vi "Individual Tube ON - OFF.vi"(6 "Single Tube ON/OFF":bool, 7 "Tube #":i32 min=0 max=63) -> ()   [LabVIEW 2020]
uses:
  <vilib>/DAQmx/write.llb/DAQmx Write (Digital U8 1Chan 1Samp).vi
  <vilib>/DAQmx/create/channels.llb/DAQmx Create Channel (DO-Digital Output).vi
  <vilib>/DAQmx/miscellaneous.llb/DAQmx Fill In Error Info.vi
panel:
  out "Status(U8) 2":u8
  out "Status(U8)":u8
  in  "lines":tag="Dev2/port0/line0:7"
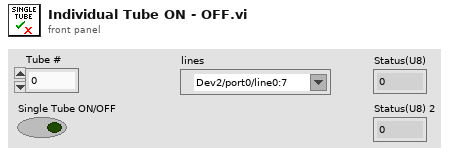
[diagram p1: front panel]
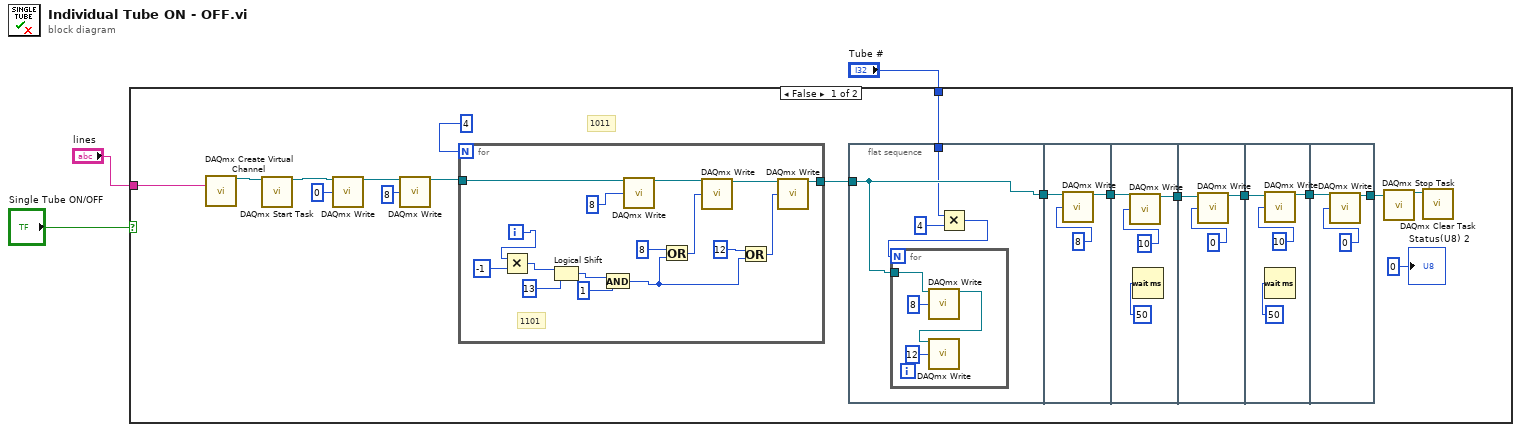
[diagram p0: block diagram]
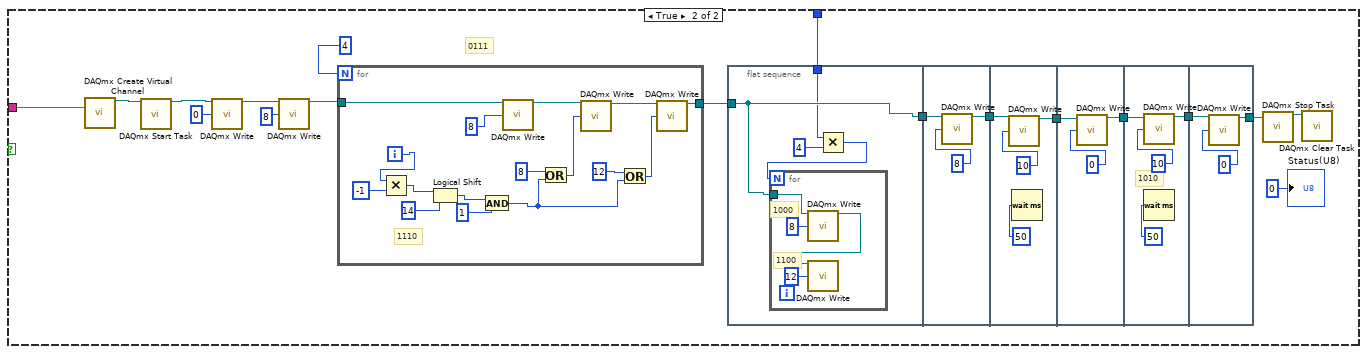
[diagram p2: hidden frame]
diagram:
  n1 = case shown="False" "Single Tube ON/OFF" {
    tunnel: "Tube #" -> [w5 w64]
    tunnel: "lines" -> [w4 w63]
    frame False {
      # "1011"
      n2 = call-poly <vilib>:"DAQmx Create Virtual Channel.vi"("lines"=w4) -> ("task out"=w16:refnum<k21>)  [unwired: 13 in, 1 out]
      n3 = call <vilib>:"DAQmx Start Task.vi"("task/channels in"=w16) -> ("task out"=w11:refnum<k21>)  [unwired: 13 in, 1 out]
      n4 = call-poly <vilib>:"DAQmx Write.vi"("task/channels in"=w11, "data"=u8 0) -> ("task out"=w10:refnum<k21>)  [unwired: 11 in, 2 out]
      n5 = call-poly <vilib>:"DAQmx Write.vi"("task/channels in"=w10, "data"=u8 8) -> ("task out"=w13:refnum<k21>)  [unwired: 11 in, 2 out]
      n6 = for {
        N: 4 -> [_]
        tunnel: w13 -> [w51]
        tunnel: [w48] -> w7
        i -> [w60]
        # "1101"
        n7 = Multiply(x=w60, y=-1) -> (x*y=w58:i32)
        n8 = Logical Shift(y=w58, x=u8 13) -> (x << y=w62:u8)
        n9 = And(x=w62, y=u32 1) -> (x .and. y?=w54:u32)
        n10 = call-poly <vilib>:"DAQmx Write.vi"("task/channels in"=w51, "data"=u32 8 ("x")) -> ("task out"=w50:refnum<k21>)  [unwired: 11 in, 2 out]
        n11 = Or(x=u32 8, y=w54) -> (x .or. y?=w55:u32)
        n12 = call-poly <vilib>:"DAQmx Write.vi"("task/channels in"=w50, "data"=w55) -> ("task out"=w49:refnum<k21>)  [unwired: 11 in, 2 out]
        n13 = Or(x=u32 12, y=w54) -> (x .or. y?=w52:u32)
        n14 = call-poly <vilib>:"DAQmx Write.vi"("task/channels in"=w49, "data"=w52) -> ("task out"=w48:refnum<k21>)  [unwired: 11 in, 2 out]
      }
      n15 = flat-sequence {
        tunnel: [w23] -> w21
        tunnel: w7 -> [w23]
        tunnel: w5 -> [w22]
        tunnel: [w30] -> w20
        tunnel: w21 -> [w31]
        tunnel: w20 -> [w34]
        tunnel: [w33] -> w19
        tunnel: w19 -> [w38]
        tunnel: [w37] -> w18
        tunnel: w18 -> [w41]
        tunnel: [w40] -> w17
        tunnel: w17 -> [w45]
        tunnel: [w44] -> w8
        frame #0 {
          n16 = Multiply(x=w22, y=4) -> (x*y=w25:i32)
          n17 = for {
            N: w25 -> [_]
            tunnel: w23 -> [w27]
            n18 = call-poly <vilib>:"DAQmx Write.vi"("task/channels in"=w27, "data"=u8 8) -> ("task out"=w26:refnum<k21>)  [unwired: 11 in, 2 out]
            n19 = call-poly <vilib>:"DAQmx Write.vi"("task/channels in"=w26, "data"=u8 12) -> ()  [unwired: 11 in, 3 out]
          }
        }
        frame #1 {
          n20 = call-poly <vilib>:"DAQmx Write.vi"("task/channels in"=w31, "data"=u8 8) -> ("task out"=w30:refnum<k21>)  [unwired: 11 in, 2 out]
        }
        frame #2 {
          n21 = call-poly <vilib>:"DAQmx Write.vi"("task/channels in"=w34, "data"=u8 10) -> ("task out"=w33:refnum<k21>)  [unwired: 11 in, 2 out]
          n22 = Wait (ms)(milliseconds to wait=u32 50) -> ()  [unwired: 1 out]
        }
        frame #3 {
          n23 = call-poly <vilib>:"DAQmx Write.vi"("task/channels in"=w38, "data"=u8 0) -> ("task out"=w37:refnum<k21>)  [unwired: 11 in, 2 out]
        }
        frame #4 {
          n24 = call-poly <vilib>:"DAQmx Write.vi"("task/channels in"=w41, "data"=u8 10) -> ("task out"=w40:refnum<k21>)  [unwired: 11 in, 2 out]
          n25 = Wait (ms)(milliseconds to wait=u32 50) -> ()  [unwired: 1 out]
        }
        frame #5 {
          n26 = call-poly <vilib>:"DAQmx Write.vi"("task/channels in"=w45, "data"=u8 0) -> ("task out"=w44:refnum<k21>)  [unwired: 11 in, 2 out]
        }
      }
      n27 = call <vilib>:"DAQmx Stop Task.vi"("task/channels in"=w8) -> ("task out"=w15:refnum<k21>)  [unwired: 13 in, 1 out]
      n28 = call <vilib>:"DAQmx Clear Task.vi"("task in"=w15) -> ()  [unwired: 14 in, 1 out]
      "Status(U8) 2" <- u8 0
    }
    frame True {
      # "0111"
      n29 = call-poly <vilib>:"DAQmx Create Virtual Channel.vi"("lines"=w63) -> ("task out"=w75:refnum<k21>)  [unwired: 13 in, 1 out]
      n30 = call <vilib>:"DAQmx Start Task.vi"("task/channels in"=w75) -> ("task out"=w70:refnum<k21>)  [unwired: 13 in, 1 out]
      n31 = call-poly <vilib>:"DAQmx Write.vi"("task/channels in"=w70, "data"=u8 0) -> ("task out"=w69:refnum<k21>)  [unwired: 11 in, 2 out]
      n32 = call-poly <vilib>:"DAQmx Write.vi"("task/channels in"=w69, "data"=u8 8) -> ("task out"=w72:refnum<k21>)  [unwired: 11 in, 2 out]
      n33 = for {
        N: 4 -> [_]
        tunnel: w72 -> [w110]
        tunnel: [w107] -> w66
        i -> [w119]
        # "1110"
        n34 = Multiply(x=w119, y=-1) -> (x*y=w117:i32)
        n35 = Logical Shift(y=w117, x=u8 14) -> (x << y=w121:u8)
        n36 = And(x=w121, y=u32 1) -> (x .and. y?=w113:u32)
        n37 = call-poly <vilib>:"DAQmx Write.vi"("task/channels in"=w110, "data"=u32 8 ("x")) -> ("task out"=w109:refnum<k21>)  [unwired: 11 in, 2 out]
        n38 = Or(x=u32 8, y=w113) -> (x .or. y?=w114:u32)
        n39 = call-poly <vilib>:"DAQmx Write.vi"("task/channels in"=w109, "data"=w114) -> ("task out"=w108:refnum<k21>)  [unwired: 11 in, 2 out]
        n40 = Or(x=u32 12, y=w113) -> (x .or. y?=w111:u32)
        n41 = call-poly <vilib>:"DAQmx Write.vi"("task/channels in"=w108, "data"=w111) -> ("task out"=w107:refnum<k21>)  [unwired: 11 in, 2 out]
      }
      n42 = flat-sequence {
        tunnel: [w82] -> w80
        tunnel: w66 -> [w82]
        tunnel: w64 -> [w81]
        tunnel: [w89] -> w79
        tunnel: w80 -> [w90]
        tunnel: w79 -> [w93]
        tunnel: [w92] -> w78
        tunnel: w78 -> [w97]
        tunnel: [w96] -> w77
        tunnel: w77 -> [w100]
        tunnel: [w99] -> w76
        tunnel: w76 -> [w104]
        tunnel: [w103] -> w67
        frame #0 {
          n43 = Multiply(x=w81, y=4) -> (x*y=w84:i32)
          n44 = for {
            N: w84 -> [_]
            tunnel: w82 -> [w86]
            # "1100"
            # "1000"
            n45 = call-poly <vilib>:"DAQmx Write.vi"("task/channels in"=w86, "data"=u8 8) -> ("task out"=w85:refnum<k21>)  [unwired: 11 in, 2 out]
            n46 = call-poly <vilib>:"DAQmx Write.vi"("task/channels in"=w85, "data"=u8 12) -> ()  [unwired: 11 in, 3 out]
          }
        }
        frame #1 {
          n47 = call-poly <vilib>:"DAQmx Write.vi"("task/channels in"=w90, "data"=u8 8) -> ("task out"=w89:refnum<k21>)  [unwired: 11 in, 2 out]
        }
        frame #2 {
          n48 = call-poly <vilib>:"DAQmx Write.vi"("task/channels in"=w93, "data"=u8 10) -> ("task out"=w92:refnum<k21>)  [unwired: 11 in, 2 out]
          n49 = Wait (ms)(milliseconds to wait=u32 50) -> ()  [unwired: 1 out]
        }
        frame #3 {
          n50 = call-poly <vilib>:"DAQmx Write.vi"("task/channels in"=w97, "data"=u8 0) -> ("task out"=w96:refnum<k21>)  [unwired: 11 in, 2 out]
        }
        frame #4 {
          # "1010"
          n51 = call-poly <vilib>:"DAQmx Write.vi"("task/channels in"=w100, "data"=u8 10) -> ("task out"=w99:refnum<k21>)  [unwired: 11 in, 2 out]
          n52 = Wait (ms)(milliseconds to wait=u32 50) -> ()  [unwired: 1 out]
        }
        frame #5 {
          n53 = call-poly <vilib>:"DAQmx Write.vi"("task/channels in"=w104, "data"=u8 0) -> ("task out"=w103:refnum<k21>)  [unwired: 11 in, 2 out]
        }
      }
      n54 = call <vilib>:"DAQmx Stop Task.vi"("task/channels in"=w67) -> ("task out"=w74:refnum<k21>)  [unwired: 13 in, 1 out]
      n55 = call <vilib>:"DAQmx Clear Task.vi"("task in"=w74) -> ()  [unwired: 14 in, 1 out]
      "Status(U8)" <- u8 0
    }
  }
